vi "Global Frame Data.vi"() -> ()   [LabVIEW 2016]
panel:
  in  "Latest Non-zero Shooter Objects Found":i32
  out "Latest Non-zero Shooter Frame Data":T1(array[cluster])
  in  "Latest Non-zero Gear Objects Found":i32
  out "Latest Non-zero Gear Frame Data":T1(array[cluster])
  in  "Gear Objects Found":i32
  out "Gear Frame Data":T1(array[cluster])
  in  "Shooter Objects Found":i32
  out "Shooter Frame Data":T1(array[cluster])
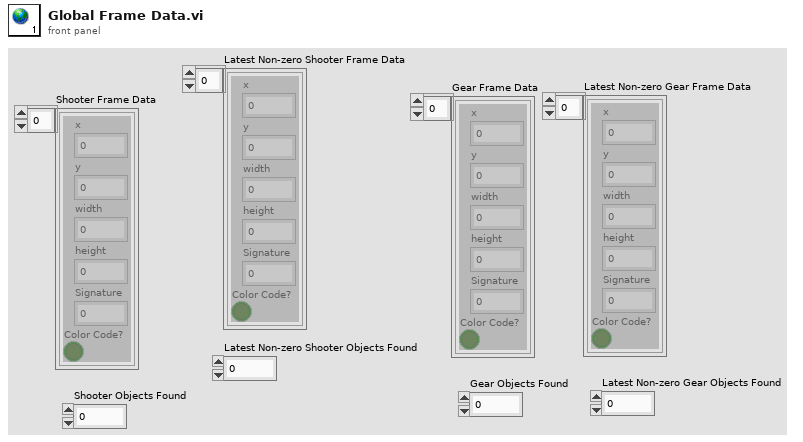
[diagram p1: front panel]
types:
  T1 = cluster{"x":u16, "y":u16, "width":u16, "height":u16, "Signature":u16, "Color Code?":bool}[]
diagram:
